vi "Scripting_ReplaceVisAndControls.vi"(0 "ViRef":refnum<vi>, 1 "OldVIsAndControls":path[](array[path]), 2 "NewVIsAndControls":path[](array[path]), 5 "error in (no error)":errorcluster) -> (15 "ReplacedVIsConPaneSize":u32[](array[numeric]), 19 "error out":errorcluster)   [LabVIEW 2012]
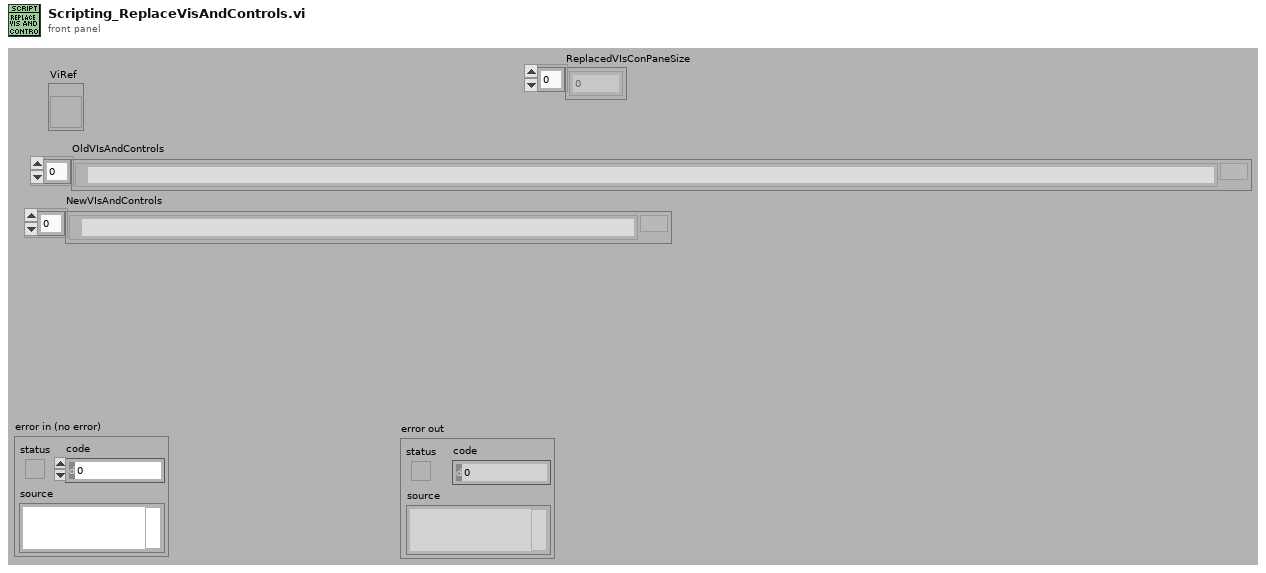
[diagram p1: front panel]
types:
  T1 = enum32{"invalid lock state", "Not Locked", "Locked (No Password)", "Password-protected"}
  T2 = cluster{"ClassControls":refnum<vi>[], "NewClassControl":path, "ReplacedVIsConPaneSize":u32[]}
  T3 = enum32{"not a typedef", "typedef", "strict typedef", "class private data"}
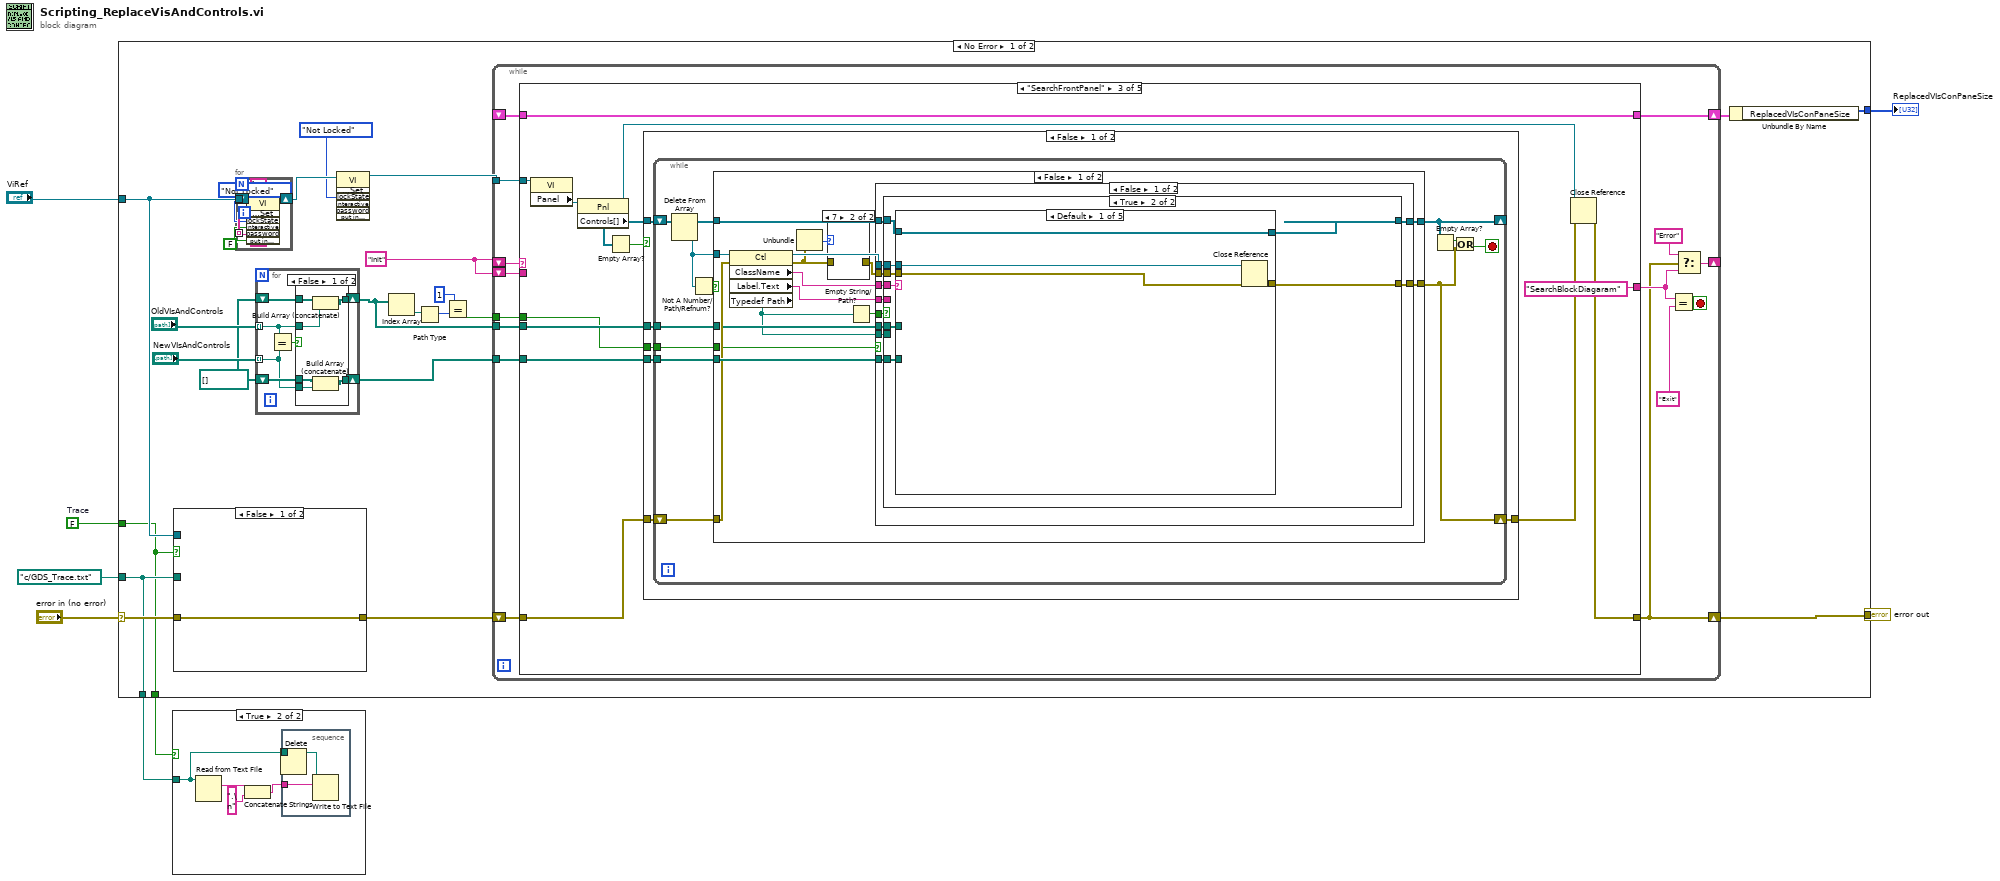
[diagram p0: block diagram]
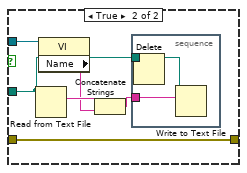
[diagram p3: hidden frame]
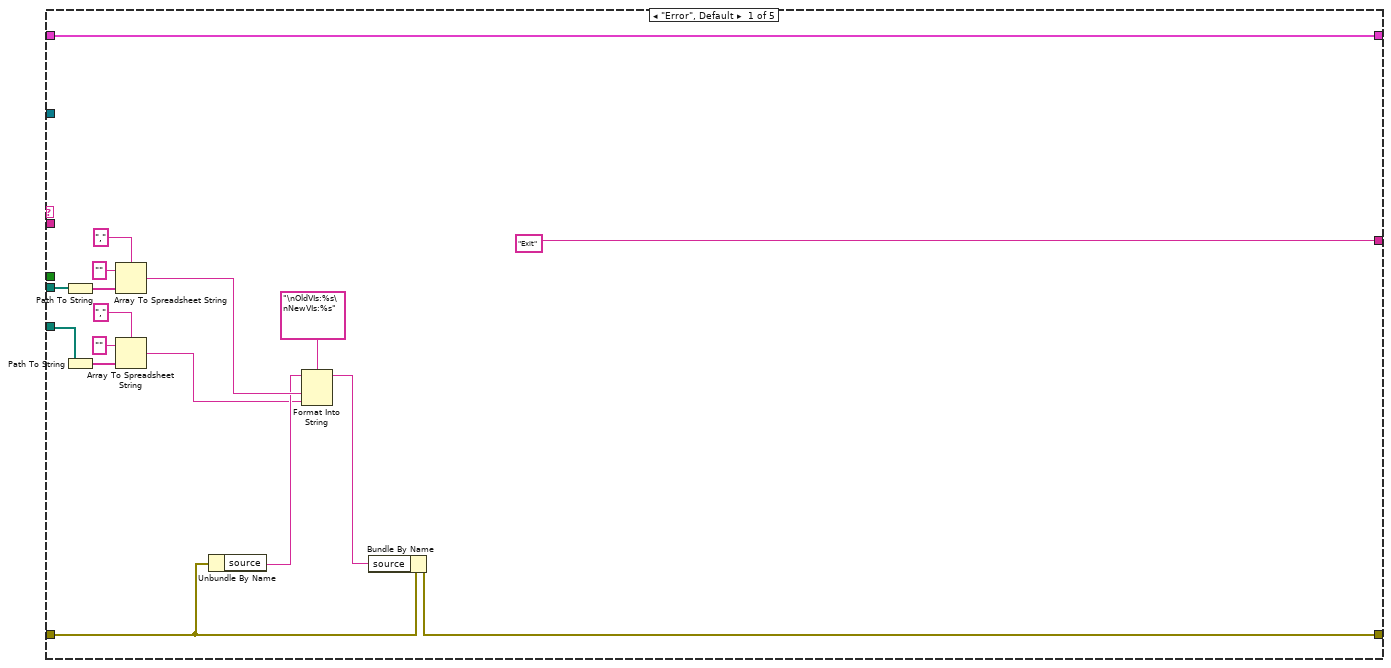
[diagram p5: hidden frame]
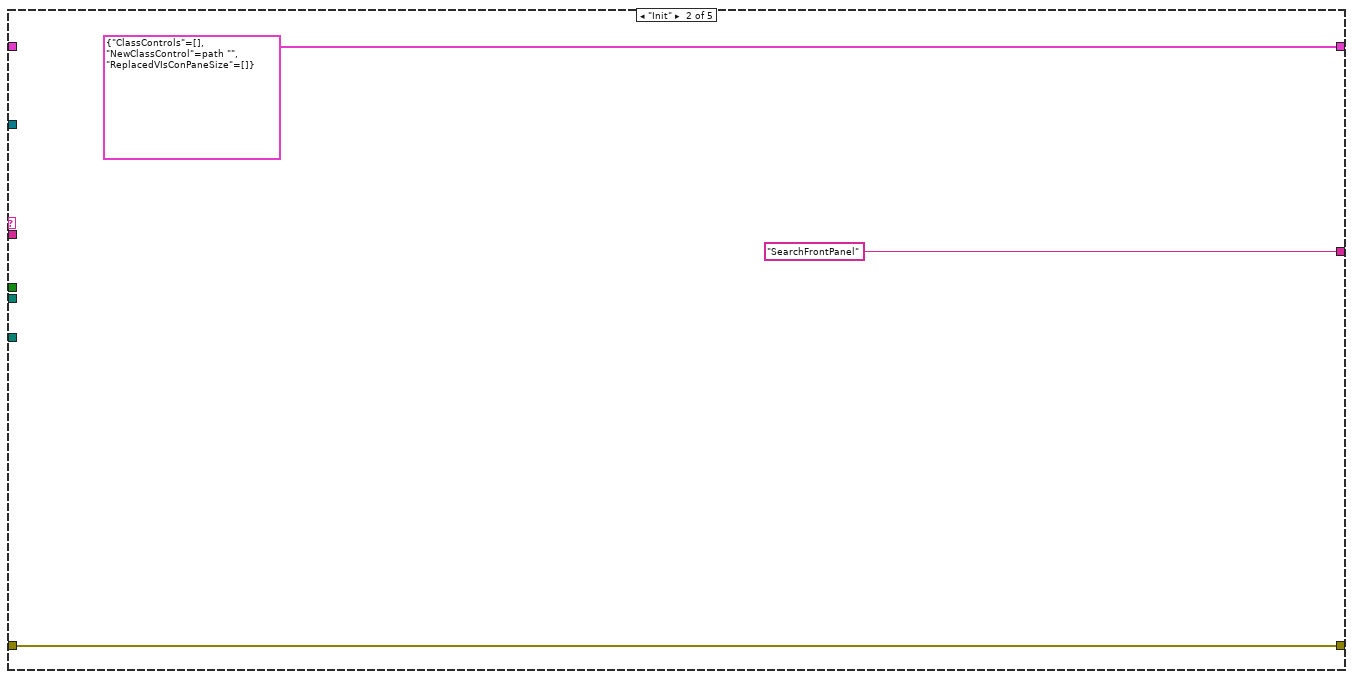
[diagram p6: hidden frame]
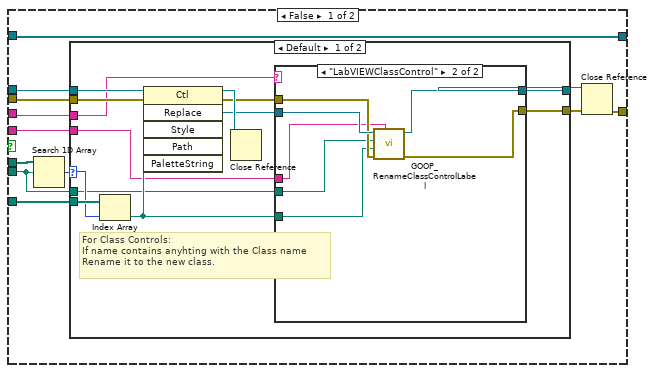
[diagram p8: hidden frame]
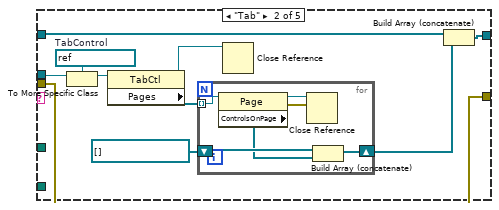
[diagram p11: hidden frame]
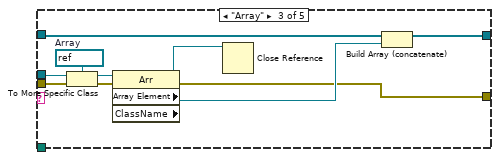
[diagram p12: hidden frame]
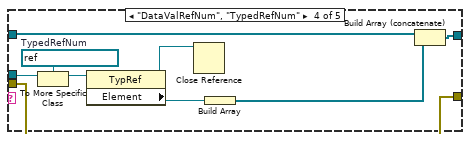
[diagram p13: hidden frame]
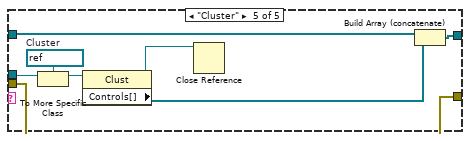
[diagram p14: hidden frame]
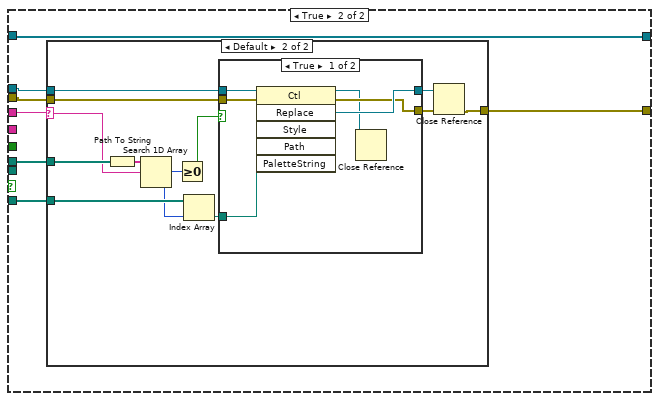
[diagram p15: hidden frame]
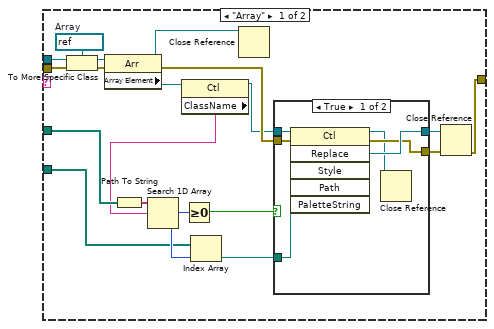
[diagram p16: hidden frame]
diagram:
  w6 = FALSE  # Trace
  n1 = case shown="No Error" "error in (no error)" {
    selector: "error in (no error)" -> [w22 w808]
    tunnel: [w30 w808] -> w8
    tunnel: "ViRef" -> [w20 _]
    tunnel: w6 -> [w18 _]
    tunnel: path "c:/GDS_Trace.txt" -> [w19 _]
    tunnel: [w19 _] -> w4
    tunnel: [w18 _] -> w3
    tunnel: [w10 _] -> w1
    frame No Error {
      w23 = path[] []
      w9 = "Init"
      n2 = case shown="False" w18 {
        tunnel: w22 -> [w31 w36]
        tunnel: [w31 w36] -> w21
        tunnel: w20 -> [_ w37]
        tunnel: w19 -> [_ w32]
        frame False {
        }
        frame True {
          n3 = Read from Text File(file (use dialog)=w32) -> (text=w35:string)  [unwired: 3 in, 3 out]
          n4 = property class="VI"(reference=w37) -> ("Name"=w34:string)  [unwired: 1 in, 2 out]
          n5 = Concatenate Strings(w35, w34) -> (w33:string)
          n6 = stacked-sequence {
            tunnel: w33 -> [w40]
            tunnel: w32 -> [w39]
            frame #0 {
              n7 = Delete(path (use dialog)=w39) -> (deleted path=w38:path)  [unwired: 4 in, 2 out]
              n8 = Write to Text File(file (use dialog)=w38, text=w40) -> ()  [unwired: 2 in, 3 out]
            }
          }
        }
      }
      n9 = for {
        tunnel: string[] ["goop rules", "i love goteborg", "Endevo Knows Goop!", "kiss"] -> [w58] mode=indexing
        shift-right: [w56] -> w28
        shift-left: w20 -> [_]
        tunnel: w20 -> [w57]
        w59 = FALSE ("Interactive")
        n10 = invoke class="VI" method="Lock State.Set"(reference=w57, "lockState"=T1."Not Locked" ("Lock State"), "interactive"=w59, "password"=w58, "put in Cache"=w59) -> (reference out=w56:refnum<vi>)  [unwired: 2 in, 6 out]
      }
      n11 = for {
        tunnel: "NewVIsAndControls" -> [w41] mode=indexing
        tunnel: "OldVIsAndControls" -> [w44] mode=indexing
        shift-right: [w45] -> w17
        shift-left: w23 -> [w46]
        shift-right: [w43] -> w13
        shift-left: w23 -> [w42]
        n12 = Equal?(x=w44, y=w41) -> (x = y?=w47:bool)
        n13 = case shown="False" w47 {
          tunnel: w46 -> [w53 w55]
          tunnel: [w52 w55] -> w45
          tunnel: w44 -> [w51 _]
          tunnel: w42 -> [w49 w54]
          tunnel: [w50 w54] -> w43
          tunnel: w41 -> [w48 _]
          frame False {
            n14 = Build Array (concatenate)(w53, w51) -> (w52:path[])
            n15 = Build Array (concatenate)(w49, w48) -> (w50:path[])
          }
          frame True {
          }
        }
      }
      n16 = invoke class="VI" method="Lock State.Set"(reference=w28, "lockState"=T1."Not Locked" ("Lock State")) -> (reference out=w26:refnum<vi>)  [unwired: 5 in, 6 out]
      n17 = Index Array(array=w17) -> (element=w14:path)  [unwired: 1 in]
      n18 = Path Type(1:w14) -> (0:w16:i16)
      n19 = Equal?(x=i16 1, y=w16) -> (x = y?=w12:bool)
      n20 = while {
        shift-right: [w68] -> w30
        shift-left: w21 -> [w75]
        shift-right: [w73] -> _
        shift-left: w9 -> [w74]
        shift-right: [w67] -> w11
        shift-left: _ -> [w66]
        tunnel: w26 -> [w63]
        tunnel: w17 -> [w65]
        tunnel: w13 -> [w64]
        tunnel: w12 -> [w62]
        shift-left: w9 -> [w61]
        stop <- w72 stop-if-true
        n21 = case shown="\"SearchFrontPanel\"" w74 {
          tunnel: w75 -> [w90 w95 w101 w310 w793]
          tunnel: [w89 w95 w100 w311 w792] -> w68
          tunnel: ["Exit" "SearchFrontPanel" "SearchBlockDiagaram" "Save" "Exit"] -> w69
          tunnel: [w91 T2 {"ClassControls"=[], "NewClassControl"=path "", "ReplacedVIsConPaneSize"=[]} w104 w304 w789] -> w67
          tunnel: w66 -> [w91 _ w104 w305 w789]
          tunnel: w63 -> [_ _ w108 w314 w794]
          tunnel: w65 -> [w88 _ w106 w309 _]
          tunnel: w64 -> [w78 _ w105 w308 _]
          tunnel: w62 -> [_ _ w96 w306 _]
          tunnel: w61 -> [_ _ _ _ _]
          frame "Error", Default {
            n22 = Path To String(path=w88) -> (string=w87:string[])
            n23 = Path To String(path=w78) -> (string=w79:string[])
            n24 = Array To Spreadsheet String(delimiter (Tab)=",", array=w87, 3:"" ("format string")) -> (spreadsheet string=w84:string)
            n25 = Array To Spreadsheet String(delimiter (Tab)=",", array=w79, 3:"" ("format string")) -> (spreadsheet string=w76:string)
            n26 = Unbundle By Name(w90) -> ("source"=w77:string)
            n27 = Format Into String(format string="\nOldVIs:%s\nNewVIs:%s", initial string=w77, w84, w76) -> (resulting string=w82:string)  [unwired: 1 in, 1 out]
            n28 = Bundle By Name(cluster=w90, "source"=w82) -> (w89:errorcluster)
          }
          frame "Init" {
          }
          frame "SearchFrontPanel" {
            n29 = property class="VI"(reference=w108) -> ("Panel"=w107:refnum<vi>)  [unwired: 1 in, 2 out]
            n30 = property class="Pnl"(reference=w107) -> (reference out=w99:refnum<vi>, "Controls[]"=w98:refnum<vi>[])  [unwired: 1 in, 1 out]
            n31 = Empty Array?(array=w98) -> (empty?=w97:bool)
            n32 = case shown="False" w97 {
              tunnel: w106 -> [w114 _]
              tunnel: w105 -> [w113 _]
              tunnel: [w112 w302] -> w102
              tunnel: w101 -> [w111 w302]
              tunnel: w98 -> [w110 _]
              tunnel: w96 -> [w109 _]
              frame False {
                n33 = while {
                  shift-right: [w118] -> _
                  shift-left: w110 -> [w126]
                  tunnel: w114 -> [w122]
                  tunnel: w113 -> [w124]
                  shift-right: [w115] -> w112
                  shift-left: w111 -> [w123]
                  tunnel: w109 -> [w119]
                  stop <- w116 stop-if-true
                  n34 = Delete From Array(array=w126) -> (deleted portion=w121:refnum<vi>, array with subset deleted=w125:refnum<vi>[])  [unwired: 2 in]
                  n35 = Not A Number/Path/Refnum?(number/path/refnum=w121) -> (NaN/Path/Refnum?=w120:bool)
                  n36 = case shown="False" w120 {
                    tunnel: w125 -> [w140 w300]
                    tunnel: [w139 w300] -> w118
                    tunnel: w124 -> [w138 _]
                    tunnel: w123 -> [w137 w301]
                    tunnel: [w136 w301] -> w115
                    tunnel: w122 -> [w135 _]
                    tunnel: w121 -> [w132 _]
                    tunnel: w119 -> [w131 _]
                    frame False {
                      n37 = property class="Ctl"(reference=w132, error in=w137) -> (reference out=w141:refnum<vi>, error out=w128:errorcluster, "ClassName"=w142:string, "Label.Text"=w130:string, "Typedef Path"=w134:path)
                      n38 = Unbundle(w128) -> ("code"=w129:i32)  [unwired: 2 out]
                      n39 = case shown="7" w129 {
                        tunnel: w128 -> [w143 _]
                        tunnel: [w143 _] -> w127
                        frame 0, Default {
                        }
                        frame 7 {
                        }
                      }
                      n40 = Empty String/Path?(string/path=w134) -> (empty?=w133:bool)
                      n41 = case shown="False" w131 {
                        tunnel: w142 -> [w154 w246]
                        tunnel: w141 -> [w153 w251]
                        tunnel: w140 -> [w152 w248]
                        tunnel: [w151 w248] -> w139
                        tunnel: w138 -> [w150 w249]
                        tunnel: w127 -> [w149 w250]
                        tunnel: [w148 w252] -> w136
                        tunnel: w135 -> [w147 w247]
                        tunnel: w134 -> [w146 _]
                        tunnel: w133 -> [w145 _]
                        tunnel: w130 -> [w144 _]
                        frame False {
                          n42 = case shown="True" w145 {
                            tunnel: w154 -> [w157 w198]
                            tunnel: w153 -> [w162 w197]
                            tunnel: w152 -> [w160 w196]
                            tunnel: [w160 w195] -> w151
                            tunnel: w150 -> [w163 w194]
                            tunnel: w149 -> [w161 w193]
                            tunnel: [w164 w192] -> w148
                            tunnel: w147 -> [w159 w191]
                            tunnel: w146 -> [w155 _]
                            tunnel: w144 -> [w156 _]
                            frame False {
                              n43 = Search 1D Array(1D array=w159, element=w155) -> (index of element=w158:i32)  [unwired: 1 in]
                              n44 = case shown="Default" w158 {
                                selector: w158 -> [w176 _]
                                tunnel: [w172 w190] -> w166
                                tunnel: [w170 w189] -> w165
                                tunnel: w163 -> [w178 _]
                                tunnel: w162 -> [w175 w190]
                                tunnel: w161 -> [w177 w189]
                                tunnel: w157 -> [w174 _]
                                tunnel: w156 -> [w167 _]
                                tunnel: w155 -> [w168 _]
                                frame Default {
                                # "For Class Controls:\nIf name contains anyhting with the Class name\nRename it to the new class."
                                n45 = Index Array(array=w178, index=w176) -> (element=w169:path)
                                n46 = invoke class="Ctl" method="Replace"(reference=w175, error in=w177, "Path"=w169) -> (reference out=w179:refnum<vi>, error out=w171:errorcluster, "Replace"=w173:refnum<vi>)  [unwired: 3 in, 3 out]
                                n47 = Close Reference(reference=w179) -> ()  [unwired: 1 in, 1 out]
                                n48 = case shown="\"LabVIEWClassControl\"" w174 {
                                tunnel: w173 -> [w181 w188]
                                tunnel: [w181 w187] -> w172
                                tunnel: w171 -> [w180 w185]
                                tunnel: [w180 w186] -> w170
                                tunnel: w169 -> [_ w184]
                                tunnel: w168 -> [_ w183]
                                tunnel: w167 -> [_ w182]
                                frame Default {
                                }
                                frame "LabVIEWClassControl" {
                                n49 = call <resource>:"GOOP_RenameClassControlLabel.vi"("Label.Text"=w182, "error in (no error)"=w185, "Path"=w184, "Typedef Path"=w183, "GObject in"=w188) -> ("error out"=w186:errorcluster, "Control out"=w187:refnum<vi>)  [unwired: 5 in]
                                }
                                }
                                }
                                frame -1 {
                                }
                              }
                              n50 = Close Reference(reference=w166, error in (no error)=w165) -> (error out=w164:errorcluster)
                            }
                            frame True {
                              n51 = case shown="Default" w198 {
                                tunnel: w197 -> [w200 w212 w228 w237 w245]
                                tunnel: w196 -> [w202 w207 w222 w234 w242]
                                tunnel: [w202 w205 w219 w233 w241] -> w195
                                tunnel: w194 -> [_ _ _ _ _]
                                tunnel: w193 -> [w199 w203 w223 w231 w239]
                                tunnel: [w201 w203 w220 w231 w239] -> w192
                                tunnel: w191 -> [_ _ _ _ _]
                                frame Default {
                                n52 = Close Reference(reference=w200, error in (no error)=w199) -> (error out=w201:errorcluster)
                                }
                                frame "Tab" {
                                w211 = refnum<vi> refnum  # TabControl
                                n53 = To More Specific Class(target class=w211, reference=w212) -> (specific class reference=w210:refnum<vi>)  [unwired: 1 in, 1 out]
                                n54 = property class="TabCtl"(reference=w210) -> (reference out=w204:refnum<vi>, "Pages"=w209:refnum<vi>[])  [unwired: 1 in, 1 out]
                                n55 = for {
                                tunnel: w209 -> [w218] mode=indexing
                                shift-right: [w217] -> w206
                                shift-left: refnum<vi>[] [] -> [w216]
                                n56 = property class="Page"(reference=w218) -> (reference out=w213:refnum<vi>, error out=w214:errorcluster, "ControlsOnPage"=w215:refnum<vi>[])  [unwired: 1 in]
                                n57 = Close Reference(reference=w213, error in (no error)=w214) -> ()  [unwired: 1 out]
                                n58 = Build Array (concatenate)(w216, w215) -> (w217:refnum<vi>[])
                                }
                                n59 = Close Reference(reference=w204) -> ()  [unwired: 1 in, 1 out]
                                n60 = Build Array (concatenate)(w207, w206) -> (w205:refnum<vi>[])
                                }
                                frame "Array" {
                                w227 = refnum<vi> refnum  # Array
                                n61 = To More Specific Class(target class=w227, reference=w228, error in=w223) -> (specific class reference=w226:refnum<vi>, error out=w224:errorcluster)
                                n62 = property class="Arr" props=["Array Element", "ClassName"](reference=w226, error in=w224) -> (reference out=w225:refnum<vi>, error out=w220:errorcluster, "Array Element"=w221:refnum<vi>)  [unwired: 1 out]
                                n63 = Close Reference(reference=w225) -> ()  [unwired: 1 in, 1 out]
                                n64 = Build Array (concatenate)(w222, w221) -> (w219:refnum<vi>[])
                                }
                                frame "DataValRefNum", "TypedRefNum" {
                                w236 = refnum<vi> refnum  # TypedRefNum
                                n65 = To More Specific Class(target class=w236, reference=w237) -> (specific class reference=w235:refnum<vi>)  [unwired: 1 in, 1 out]
                                n66 = property class="TypRef"(reference=w235) -> (reference out=w232:refnum<vi>, "Element"=w230:refnum<vi>)  [unwired: 1 in, 1 out]
                                n67 = Close Reference(reference=w232) -> ()  [unwired: 1 in, 1 out]
                                n68 = Build Array(w230) -> (w229:refnum<vi>[])
                                n69 = Build Array (concatenate)(w234, w229) -> (w233:refnum<vi>[])
                                }
                                frame "Cluster" {
                                w244 = refnum<vi> refnum  # Cluster
                                n70 = To More Specific Class(target class=w244, reference=w245) -> (specific class reference=w243:refnum<vi>)  [unwired: 1 in, 1 out]
                                n71 = property class="Clust"(reference=w243) -> (reference out=w240:refnum<vi>, "Controls[]"=w238:refnum<vi>[])  [unwired: 1 in, 1 out]
                                n72 = Close Reference(reference=w240) -> ()  [unwired: 1 in, 1 out]
                                n73 = Build Array (concatenate)(w242, w238) -> (w241:refnum<vi>[])
                                }
                              }
                            }
                          }
                        }
                        frame True {
                          n74 = case shown="Default" w246 {
                            selector: w246 -> [_ w280]
                            tunnel: [w256 w289] -> w252
                            tunnel: w251 -> [w259 w288]
                            tunnel: w250 -> [w260 w287]
                            tunnel: w249 -> [w258 w286]
                            tunnel: w247 -> [w257 w284]
                            frame "Array" {
                              w271 = refnum<vi> refnum  # Array
                              n75 = To More Specific Class(target class=w271, reference=w259, error in=w260) -> (specific class reference=w270:refnum<vi>, error out=w261:errorcluster)
                              n76 = property class="Arr"(reference=w270, error in=w261) -> (reference out=w269:refnum<vi>, error out=w262:errorcluster, "Array Element"=w255:refnum<vi>)
                              n77 = Path To String(path=w257) -> (string=w265:string[])
                              n78 = property class="Ctl"(reference=w255) -> (reference out=w254:refnum<vi>, "ClassName"=w253:string)  [unwired: 1 in, 1 out]
                              n79 = Search 1D Array(1D array=w265, element=w253) -> (index of element=w263:i32)  [unwired: 1 in]
                              n80 = Greater Or Equal To 0?(x=w263) -> (x >= 0?=w264:bool)
                              n81 = Index Array(array=w258, index=w263) -> (element=w266:path)
                              n82 = Close Reference(reference=w269) -> ()  [unwired: 1 in, 1 out]
                              n83 = case shown="True" w264 {
                                tunnel: [w277 w279] -> w268
                                tunnel: [w276 w278] -> w267
                                tunnel: w254 -> [w274 w279]
                                tunnel: w262 -> [w273 w278]
                                tunnel: w266 -> [w272 _]
                                frame True {
                                n84 = invoke class="Ctl" method="Replace"(reference=w274, error in=w273, "Path"=w272) -> (reference out=w275:refnum<vi>, error out=w276:errorcluster, "Replace"=w277:refnum<vi>)  [unwired: 3 in, 3 out]
                                n85 = Close Reference(reference=w275) -> ()  [unwired: 1 in, 1 out]
                                }
                                frame False {
                                }
                              }
                              n86 = Close Reference(reference=w268, error in (no error)=w267) -> (error out=w256:errorcluster)
                            }
                            frame Default {
                              n87 = Path To String(path=w284) -> (string=w283:string[])
                              n88 = Search 1D Array(1D array=w283, element=w280) -> (index of element=w281:i32)  [unwired: 1 in]
                              n89 = Greater Or Equal To 0?(x=w281) -> (x >= 0?=w282:bool)
                              n90 = Index Array(array=w286, index=w281) -> (element=w285:path)
                              n91 = case shown="True" w282 {
                                tunnel: [w297 w299] -> w291
                                tunnel: [w296 w298] -> w290
                                tunnel: w288 -> [w294 w299]
                                tunnel: w287 -> [w293 w298]
                                tunnel: w285 -> [w292 _]
                                frame True {
                                n92 = invoke class="Ctl" method="Replace"(reference=w294, error in=w293, "Path"=w292) -> (reference out=w295:refnum<vi>, error out=w296:errorcluster, "Replace"=w297:refnum<vi>)  [unwired: 3 in, 3 out]
                                n93 = Close Reference(reference=w295) -> ()  [unwired: 1 in, 1 out]
                                }
                                frame False {
                                }
                              }
                              n94 = Close Reference(reference=w291, error in (no error)=w290) -> (error out=w289:errorcluster)
                            }
                          }
                        }
                      }
                    }
                    frame True {
                    }
                  }
                  n95 = Empty Array?(array=w118) -> (empty?=w117:bool)
                  n96 = Or(x=w117, y=w115) -> (x .or. y?=w116:bool)
                }
              }
              frame True {
              }
            }
            n97 = Close Reference(reference=w99, error in (no error)=w102) -> (error out=w100:errorcluster)
          }
          frame "SearchBlockDiagaram" {
            n98 = property class="VI"(reference=w314) -> (error out=w307:errorcluster, "Diagram"=w313:refnum<vi>)  [unwired: 1 in, 1 out]
            n99 = case shown="No Error" w307 {
              tunnel: w313 -> [w324 w787]
              tunnel: [w322 w788] -> w311
              tunnel: w310 -> [w321 w788]
              tunnel: w309 -> [w320 _]
              tunnel: w308 -> [w319 _]
              tunnel: w306 -> [w317 _]
              tunnel: [w315 _] -> w303
              frame No Error {
                n100 = property class="TopLvlDiag"(reference=w324) -> (reference out=w318:refnum<vi>, "AllObjs[]"=w323:refnum<vi>[])  [unwired: 1 in, 1 out]
                n101 = while {
                  shift-right: [w337] -> _
                  shift-left: w323 -> [w341]
                  shift-right: [w326] -> w322
                  shift-left: w321 -> [w335]
                  tunnel: w320 -> [w334]
                  tunnel: w319 -> [w333]
                  tunnel: w317 -> [w330]
                  shift-right: [w328] -> w315
                  shift-left: u32[] [] -> [w329]
                  stop <- w339 stop-if-true
                  # "LabVIEWClassConstant"
                  n102 = Delete From Array(array=w341) -> (deleted portion=w332:refnum<vi>, array with subset deleted=w338:refnum<vi>[])  [unwired: 2 in]
                  n103 = Not A Number/Path/Refnum?(number/path/refnum=w332) -> (NaN/Path/Refnum?=w331:bool)
                  n104 = case shown="False" w331 {
                    tunnel: [w355 _] -> w336
                    tunnel: [w352 w786] -> w327
                    tunnel: w335 -> [w351 w786]
                    tunnel: w334 -> [w350 _]
                    tunnel: w333 -> [w349 _]
                    tunnel: w332 -> [w348 _]
                    tunnel: w330 -> [w347 _]
                    tunnel: w329 -> [w346 w785]
                    tunnel: [w345 w785] -> w328
                    frame False {
                      n105 = property class="GObj"(reference=w348, error in=w351) -> (reference out=w357:refnum<vi>, error out=w358:errorcluster, "Class Name"=w356:string)
                      n106 = case shown="False" w347 {
                        tunnel: w358 -> [w368 w735]
                        tunnel: w357 -> [w367 w738]
                        tunnel: w356 -> [w366 w732]
                        tunnel: [w365 _] -> w355
                        tunnel: [w364 w736] -> w354
                        tunnel: [w363 w737] -> w353
                        tunnel: w350 -> [w362 w733]
                        tunnel: w349 -> [w361 w739]
                        tunnel: w346 -> [w360 w731]
                        tunnel: [w359 w731] -> w345
                        frame False {
                          n107 = case shown="Default" w366 {
                            selector: w366 -> [w378 _ _ _ _ _ _ _ _ _]
                            tunnel: w367 -> [w376 w589 w609 w629 w649 w669 w688 w707 w718 w730]
                            tunnel: w368 -> [w377 w584 w604 w626 w646 w666 w687 w703 w714 w726]
                            tunnel: [w371 w582 w602 w619 w640 w662 w680 w699 w710 w721] -> w364
                            tunnel: [w372 w580 w600 w621 w641 w660 w679 w701 w712 w724] -> w365
                            tunnel: [w373 w583 w603 w620 w639 w661 w681 w700 w711 w723] -> w363
                            tunnel: w362 -> [w375 _ _ _ _ _ _ _ _ _]
                            tunnel: w361 -> [w374 _ _ _ _ _ _ _ _ _]
                            tunnel: w360 -> [w370 w578 w598 w618 w638 w658 w678 w697 w708 w719]
                            tunnel: [w369 w578 w598 w618 w638 w658 w678 w697 w708 w719] -> w359
                            frame Default {
                              n108 = case shown="\"PolymorphicSubVI\", \"SubVI\"" w378 {
                                selector: w378 -> [w380 _ _ _ _]
                                tunnel: w377 -> [w383 w467 w503 w522 w555]
                                tunnel: w376 -> [w385 w468 w504 w532 w564]
                                tunnel: [w387 w466 w502 w531 w563] -> w371
                                tunnel: [w384 w465 w501 w530 w562] -> w373
                                tunnel: w375 -> [w382 w459 w495 w526 w558]
                                tunnel: w374 -> [w381 w456 w492 w523 w556]
                                tunnel: [_ _ _ w515 w547] -> w372
                                tunnel: w370 -> [w379 w455 w491 w514 w546]
                                tunnel: [w379 w454 w491 w514 w546] -> w369
                                frame Default {
                                w389 = refnum<vi> refnum  # Constant
                                n109 = To More Specific Class(target class=w389, reference=w385, error in=w383) -> (specific class reference=w388:refnum<vi>, error out=w386:errorcluster)
                                n110 = case shown="Error" w386 {
                                selector: w386 -> [w399 _]
                                tunnel: w388 -> [w395 _]
                                tunnel: [w400 w452] -> w387
                                tunnel: w385 -> [w393 w453]
                                tunnel: [w398 w453] -> w384
                                tunnel: w383 -> [w394 w452]
                                tunnel: w382 -> [w392 _]
                                tunnel: w381 -> [w390 _]
                                tunnel: w380 -> [w396 _]
                                frame No Error {
                                n111 = case shown="Default" w396 {
                                tunnel: w395 -> [_ w447]
                                tunnel: w399 -> [w419 w446]
                                tunnel: [w412 w445] -> w397
                                tunnel: w393 -> [w420 _]
                                tunnel: w392 -> [w418 w444]
                                tunnel: [w413 w443] -> w391
                                frame "LabVIEWClassConstant" {
                                w421 = refnum<vi> refnum  # LabVIEWClassConstant
                                n112 = for {
                                tunnel: w418 -> [w440] mode=indexing
                                tunnel: [w439] -> w417 mode=indexing
                                n113 = Strip Path(path=w440) -> (name=w439:string)  [unwired: 1 out]
                                }
                                n114 = To More Specific Class(target class=w421, reference=w420, error in=w419) -> (specific class reference=w423:refnum<vi>, error out=w422:errorcluster)
                                n115 = disable-structure shown="Enabled" {
                                disable-tunnel: w423 -> [w430 _]
                                disable-tunnel: w422 -> [w429 w438]
                                disable-tunnel: [w428 "-1"] -> w414
                                disable-tunnel: [w424 w438] -> w412
                                frame Enabled {
                                n116 = property class="LVClassConstant"(reference=w430, error in=w429) -> (error out=w424:errorcluster, "Value"=w431:variant)  [unwired: 1 out]
                                n117 = Flatten To String(anything=w431) -> (data string=w432:string)  [unwired: 3 in, 2 out]
                                n118 = Match Pattern(string=w432, regular expression="[~\\00\\01\\02\\03\\04\\05\\06\\07\\08\\09\\0A\\0B\\0C\\0D\\0E\\0F\\10\\11\\12\\13\\14\\15\\16\\17\\18\\19\\1A\\1B\\1C\\1D\\1E]+\\.lvclass") -> (match substring=w426:string)  [unwired: 1 in, 3 out]
                                n119 = Match Pattern(string=w426, regular expression="[~A-Za-zäöåÄÖÅÜü_]*") -> (after substring=w425:string)  [unwired: 1 in, 3 out]
                                n120 = Match Pattern(string=w425, regular expression="\\.lvclass") -> (before substring=w436:string)  [unwired: 1 in, 3 out]
                                n121 = Format Into String(format string="%s.ctl", w436) -> (resulting string=w428:string)  [unwired: 2 in, 1 out]
                                }
                                frame Disabled {
                                }
                                }
                                n122 = To Lower Case(string=w417) -> (all lower case string=w416:string[])
                                n123 = To Lower Case(string=w414) -> (all lower case string=w415:string)
                                n124 = Search 1D Array(1D array=w416, element=w415) -> (index of element=w413:i32)  [unwired: 1 in]
                                }
                                frame Default {
                                n125 = property class="Const"(reference=w447, error in=w446) -> (error out=w445:errorcluster, "Typedef Path"=w442:path)  [unwired: 1 out]
                                n126 = Empty String/Path?(string/path=w442) -> (empty?=w441:bool)
                                n127 = case shown="False" w441 {
                                tunnel: w444 -> [w450 _]
                                tunnel: [w449 -1 ("index of element")] -> w443
                                tunnel: w442 -> [w448 _]
                                frame False {
                                n128 = Search 1D Array(1D array=w450, element=w448) -> (index of element=w449:i32)  [unwired: 1 in]
                                }
                                frame True {
                                }
                                }
                                }
                                }
                                n129 = case shown="0, Default" w391 {
                                selector: w391 -> [w407 _]
                                tunnel: w394 -> [w408 w410]
                                tunnel: w395 -> [w409 w411]
                                tunnel: [w403 w411] -> w398
                                tunnel: [w402 w410] -> w400
                                tunnel: w390 -> [w406 _]
                                tunnel: w397 -> [_ _]
                                tunnel: [w401 _] -> _
                                frame 0, Default {
                                n130 = Index Array(array=w406, index=w407) -> (element=w405:path)
                                n131 = invoke class="Const" method="Replace"(reference=w409, error in=w408, "Path"=w405) -> (reference out=w404:refnum<vi>, error out=w402:errorcluster, "Replace"=w403:refnum<vi>)  [unwired: 3 in, 3 out]
                                n132 = Close Reference(reference=w404) -> (error out=w401:errorcluster)  [unwired: 1 in]
                                }
                                frame -1 {
                                }
                                }
                                }
                                frame Error {
                                }
                                }
                                }
                                frame "PolymorphicSubVI", "SubVI" {
                                n133 = To More Specific Class(target class=refnum<vi> refnum ("WhileLoop"), reference=w468, error in=w467) -> (specific class reference=w463:refnum<vi>, error out=w462:errorcluster)
                                n134 = property class="SubVI"(reference=w463, error in=w462) -> (reference out=w460:refnum<vi>, error out=w461:errorcluster, "VI Path"=w458:path)
                                n135 = Search 1D Array(1D array=w459, element=w458) -> (index of element=w457:i32)  [unwired: 1 in]
                                n136 = case shown="0, Default" w457 {
                                selector: w457 -> [w487 _]
                                tunnel: w461 -> [w484 w489]
                                tunnel: w460 -> [w485 w490]
                                tunnel: [w480 w490] -> w465
                                tunnel: [w479 w489] -> w466
                                tunnel: w456 -> [w486 _]
                                tunnel: [w473 _] -> _
                                tunnel: w455 -> [w471 w488]
                                tunnel: [w469 w488] -> w454
                                frame 0, Default {
                                n137 = Index Array(array=w486, index=w487) -> (element=w483:path)
                                n138 = call <resource>:"Scripting_ReplaceSubVI.vi"("error in"=w484, "NewVIToReplaceWith"=w483, "CurrentSubVI"=w485) -> ("error out"=w479:errorcluster, "ReplacedObject(SubVI)"=w480:refnum<vi>)  [unwired: 7 in]
                                n139 = To More Specific Class(target class=refnum<vi> refnum ("WhileLoop"), reference=w480, error in=w479) -> (specific class reference=w478:refnum<vi>, error out=w477:errorcluster)
                                n140 = property class="SubVI"(reference=w478, error in=w477) -> ("VI Ref"=w476:refnum<vi>)  [unwired: 2 out]
                                n141 = property class="VI" props=["Exec.State", "ConPane"](reference=w476) -> (reference out=w472:refnum<vi>, "ConPane"=w482:refnum<vi>)  [unwired: 1 in, 2 out]
                                n142 = property class="ConPane"(reference=w482) -> (reference out=w474:refnum<vi>, error out=w475:errorcluster, "NumConns"=w470:u32)  [unwired: 1 in]
                                n143 = Build Array (concatenate)(w471, w470) -> (w469:u32[])
                                n144 = Close Reference(reference=w474, error in (no error)=w475) -> (error out=w473:errorcluster)
                                n145 = Close Reference(reference=w472, error in (no error)=w473) -> ()  [unwired: 1 out]
                                }
                                frame -1 {
                                }
                                }
                                }
                                frame "StaticVIReference" {
                                n146 = To More Specific Class(target class=refnum<vi> refnum ("WhileLoop"), reference=w504, error in=w503) -> (specific class reference=w499:refnum<vi>, error out=w498:errorcluster)
                                n147 = property class="StatVIRef"(reference=w499, error in=w498) -> (reference out=w496:refnum<vi>, error out=w497:errorcluster, "Path"=w494:path)
                                n148 = Search 1D Array(1D array=w495, element=w494) -> (index of element=w493:i32)  [unwired: 1 in]
                                n149 = case shown="-1" w493 {
                                selector: w493 -> [w511 _]
                                tunnel: w497 -> [w508 w512]
                                tunnel: w496 -> [w509 w513]
                                tunnel: [w506 w513] -> w501
                                tunnel: [w505 w512] -> w502
                                tunnel: w492 -> [w510 _]
                                frame 0, Default {
                                n150 = Index Array(array=w510, index=w511) -> (element=w507:path)
                                n151 = property class="StatVIRef"(reference=w509, error in=w508, "Path"=w507) -> (reference out=w506:refnum<vi>, error out=w505:errorcluster)
                                }
                                frame -1 {
                                }
                                }
                                }
                                frame "ClusterConstant" {
                                n152 = To More Specific Class(target class=refnum<vi> refnum ("WhileLoop"), reference=w532, error in=w522) -> (specific class reference=w528:refnum<vi>, error out=w527:errorcluster)
                                n153 = property class="ClustCnst"(reference=w528, error in=w527) -> (reference out=w520:refnum<vi>, error out=w519:errorcluster, "Typedef Path"=w525:path)
                                n154 = Search 1D Array(1D array=w526, element=w525) -> (index of element=w524:i32)  [unwired: 1 in]
                                n155 = property class="ClustCnst"(reference=w520, error in=w519) -> (reference out=w518:refnum<vi>, "Elements[]"=w516:refnum<vi>[], "Typedef?"=w521:T3)  [unwired: 1 out]
                                n156 = Not Equal To 0?(x=w521) -> (x != 0?=w517:bool)
                                n157 = case shown="True" w517 {
                                tunnel: [w533 _] -> w515
                                tunnel: w516 -> [w533 w534]
                                frame False {
                                }
                                frame True {
                                n158 = for {
                                tunnel: w534 -> [w535] mode=indexing
                                n159 = Close Reference(reference=w535) -> ()  [unwired: 1 in, 1 out]
                                }
                                }
                                }
                                n160 = case shown="0, Default" w524 {
                                selector: w524 -> [w541 _]
                                tunnel: w522 -> [w542 w544]
                                tunnel: w518 -> [w543 w545]
                                tunnel: [w537 w545] -> w530
                                tunnel: [w536 w544] -> w531
                                tunnel: w523 -> [w540 _]
                                frame 0, Default {
                                n161 = Index Array(array=w540, index=w541) -> (element=w539:path)
                                n162 = invoke class="ClustCnst" method="Replace"(reference=w543, error in=w542, "Path"=w539) -> (reference out=w538:refnum<vi>, error out=w536:errorcluster, "Replace"=w537:refnum<vi>)  [unwired: 3 in, 3 out]
                                n163 = Close Reference(reference=w538) -> ()  [unwired: 1 in, 1 out]
                                }
                                frame -1 {
                                }
                                }
                                }
                                frame "ArrayConstant" {
                                n164 = To More Specific Class(target class=refnum<vi> refnum ("WhileLoop"), reference=w564, error in=w555) -> (specific class reference=w560:refnum<vi>, error out=w559:errorcluster)
                                n165 = property class="ArrCnst"(reference=w560, error in=w559) -> (reference out=w550:refnum<vi>, error out=w551:errorcluster, "Typedef Path"=w557:path)
                                n166 = Search 1D Array(1D array=w558, element=w557) -> (index of element=w548:i32)  [unwired: 1 in]
                                n167 = property class="ArrCnst"(reference=w550, error in=w551) -> (reference out=w549:refnum<vi>, "Element"=w552:refnum<vi>, "Typedef?"=w554:T3)  [unwired: 1 out]
                                n168 = Not Equal To 0?(x=w554) -> (x != 0?=w553:bool)
                                n169 = case shown="False" w553 {
                                tunnel: w552 -> [w566 w567]
                                tunnel: [w565 _] -> w547
                                frame False {
                                n170 = Build Array(w566) -> (w565:refnum<vi>[])
                                }
                                frame True {
                                n171 = Close Reference(reference=w567) -> ()  [unwired: 1 in, 1 out]
                                }
                                }
                                n172 = case shown="0, Default" w548 {
                                selector: w548 -> [w573 _]
                                tunnel: w555 -> [w574 w576]
                                tunnel: w549 -> [w575 w577]
                                tunnel: [w569 w577] -> w562
                                tunnel: [w568 w576] -> w563
                                tunnel: w556 -> [w572 _]
                                frame 0, Default {
                                n173 = Index Array(array=w572, index=w573) -> (element=w571:path)
                                n174 = invoke class="ArrCnst" method="Replace"(reference=w575, error in=w574, "Path"=w571) -> (reference out=w570:refnum<vi>, error out=w568:errorcluster, "Replace"=w569:refnum<vi>)  [unwired: 3 in, 3 out]
                                n175 = Close Reference(reference=w570) -> ()  [unwired: 1 in, 1 out]
                                }
                                frame -1 {
                                }
                                }
                                }
                              }
                            }
                            frame "CaseSelector", "CaseStructure" {
                              n176 = To More Specific Class(target class=refnum<vi> refnum ("CaseSelector"), reference=w589, error in=w584) -> (specific class reference=w587:refnum<vi>, error out=w585:errorcluster)
                              n177 = property class="CaseSel"(reference=w587, error in=w585) -> (reference out=w583:refnum<vi>, error out=w581:errorcluster, "Frames[]"=w586:refnum<vi>[])
                              n178 = for {
                                tunnel: w586 -> [w597] mode=indexing
                                shift-right: [w590] -> w582
                                shift-left: w581 -> [w596]
                                shift-right: [w593] -> w580
                                shift-left: refnum<vi>[] [] -> [w595]
                                n179 = property class="Diag"(reference=w597, error in=w596) -> (reference out=w591:refnum<vi>, error out=w592:errorcluster, "AllObjs[]"=w594:refnum<vi>[])
                                n180 = Build Array (concatenate)(w595, w594) -> (w593:refnum<vi>[])
                                n181 = Close Reference(reference=w591, error in (no error)=w592) -> (error out=w590:errorcluster)
                              }
                            }
                            frame "DisableStructure" {
                              n182 = To More Specific Class(target class=refnum<vi> refnum ("CaseSelector"), reference=w609, error in=w604) -> (specific class reference=w607:refnum<vi>, error out=w605:errorcluster)
                              n183 = property class="DisableStructure"(reference=w607, error in=w605) -> (reference out=w603:refnum<vi>, error out=w601:errorcluster, "Frames[]"=w606:refnum<vi>[])
                              n184 = for {
                                tunnel: w606 -> [w617] mode=indexing
                                shift-right: [w610] -> w602
                                shift-left: w601 -> [w616]
                                shift-right: [w613] -> w600
                                shift-left: refnum<vi>[] [] -> [w615]
                                n185 = property class="Diag"(reference=w617, error in=w616) -> (reference out=w611:refnum<vi>, error out=w612:errorcluster, "AllObjs[]"=w614:refnum<vi>[])
                                n186 = Build Array (concatenate)(w615, w614) -> (w613:refnum<vi>[])
                                n187 = Close Reference(reference=w611, error in (no error)=w612) -> (error out=w610:errorcluster)
                              }
                            }
                            frame "MultiFrameStructure" {
                              (unwired) string[] []
                              n188 = To More Specific Class(target class=refnum<vi> refnum ("MultiFrameStructure"), reference=w629, error in=w626) -> (specific class reference=w628:refnum<vi>, error out=w627:errorcluster)
                              n189 = property class="MFStruct"(reference=w628, error in=w627) -> (reference out=w620:refnum<vi>, error out=w623:errorcluster, "Frames[]"=w622:refnum<vi>[])
                              n190 = for {
                                tunnel: w622 -> [w637] mode=indexing
                                shift-right: [w630] -> w619
                                shift-left: w623 -> [w636]
                                shift-right: [w633] -> w621
                                shift-left: refnum<vi>[] [] -> [w635]
                                n191 = property class="Diag"(reference=w637, error in=w636) -> (reference out=w631:refnum<vi>, error out=w632:errorcluster, "AllObjs[]"=w634:refnum<vi>[])
                                n192 = Build Array (concatenate)(w635, w634) -> (w633:refnum<vi>[])
                                n193 = Close Reference(reference=w631, error in (no error)=w632) -> (error out=w630:errorcluster)
                              }
                            }
                            frame "EventStructure" {
                              n194 = To More Specific Class(target class=refnum<vi> refnum ("EventStructure"), reference=w649, error in=w646) -> (specific class reference=w648:refnum<vi>, error out=w647:errorcluster)
                              n195 = property class="EvntStruct"(reference=w648, error in=w647) -> (reference out=w639:refnum<vi>, error out=w643:errorcluster, "Frames[]"=w642:refnum<vi>[])
                              n196 = for {
                                tunnel: w642 -> [w657] mode=indexing
                                shift-right: [w650] -> w640
                                shift-left: w643 -> [w656]
                                shift-right: [w653] -> w641
                                shift-left: refnum<vi>[] [] -> [w655]
                                n197 = property class="Diag"(reference=w657, error in=w656) -> (reference out=w651:refnum<vi>, error out=w652:errorcluster, "AllObjs[]"=w654:refnum<vi>[])
                                n198 = Build Array (concatenate)(w655, w654) -> (w653:refnum<vi>[])
                                n199 = Close Reference(reference=w651, error in (no error)=w652) -> (error out=w650:errorcluster)
                              }
                            }
                            frame "Sequence" {
                              n200 = To More Specific Class(target class=refnum<vi> refnum ("Sequence"), reference=w669, error in=w666) -> (specific class reference=w668:refnum<vi>, error out=w667:errorcluster)
                              n201 = property class="Seq"(reference=w668, error in=w667) -> (reference out=w661:refnum<vi>, error out=w663:errorcluster, "Frames[]"=w659:refnum<vi>[])
                              n202 = for {
                                tunnel: w659 -> [w677] mode=indexing
                                shift-right: [w670] -> w662
                                shift-left: w663 -> [w676]
                                shift-right: [w673] -> w660
                                shift-left: refnum<vi>[] [] -> [w675]
                                n203 = property class="Diag"(reference=w677, error in=w676) -> (reference out=w671:refnum<vi>, error out=w672:errorcluster, "AllObjs[]"=w674:refnum<vi>[])
                                n204 = Build Array (concatenate)(w675, w674) -> (w673:refnum<vi>[])
                                n205 = Close Reference(reference=w671, error in (no error)=w672) -> (error out=w670:errorcluster)
                              }
                            }
                            frame "FlatSequence" {
                              n206 = To More Specific Class(target class=refnum<vi> refnum ("FlatSequence"), reference=w688, error in=w687) -> (specific class reference=w685:refnum<vi>)  [unwired: 1 out]
                              n207 = property class="FlatSeq"(reference=w685) -> (reference out=w681:refnum<vi>, error out=w683:errorcluster, "Diagrams[]"=w682:refnum<vi>[])  [unwired: 1 in]
                              n208 = for {
                                tunnel: w682 -> [w696] mode=indexing
                                shift-right: [w689] -> w680
                                shift-left: w683 -> [w695]
                                shift-right: [w692] -> w679
                                shift-left: refnum<vi>[] [] -> [w694]
                                n209 = property class="Diag"(reference=w696, error in=w695) -> (reference out=w690:refnum<vi>, error out=w691:errorcluster, "AllObjs[]"=w693:refnum<vi>[])
                                n210 = Build Array (concatenate)(w694, w693) -> (w692:refnum<vi>[])
                                n211 = Close Reference(reference=w690, error in (no error)=w691) -> (error out=w689:errorcluster)
                              }
                            }
                            frame "WhileLoop" {
                              n212 = To More Specific Class(target class=refnum<vi> refnum ("WhileLoop"), reference=w707, error in=w703) -> (specific class reference=w706:refnum<vi>, error out=w704:errorcluster)
                              n213 = property class="WLoop"(reference=w706, error in=w704) -> (reference out=w700:refnum<vi>, error out=w699:errorcluster, "Diagram"=w702:refnum<vi>)
                              n214 = property class="Diag"(reference=w702) -> (reference out=w698:refnum<vi>, "AllObjs[]"=w701:refnum<vi>[])  [unwired: 1 in, 1 out]
                              n215 = Close Reference(reference=w698) -> ()  [unwired: 1 in, 1 out]
                            }
                            frame "TimedLoop" {
                              n216 = To More Specific Class(target class=refnum<vi> refnum ("WhileLoop"), reference=w718, error in=w714) -> (specific class reference=w717:refnum<vi>, error out=w715:errorcluster)
                              n217 = property class="WLoop"(reference=w717, error in=w715) -> (reference out=w711:refnum<vi>, error out=w710:errorcluster, "Diagram"=w713:refnum<vi>)
                              n218 = property class="Diag"(reference=w713) -> (reference out=w709:refnum<vi>, "AllObjs[]"=w712:refnum<vi>[])  [unwired: 1 in, 1 out]
                              n219 = Close Reference(reference=w709) -> ()  [unwired: 1 in, 1 out]
                            }
                            frame "ForLoop" {
                              n220 = To More Specific Class(target class=refnum<vi> refnum ("WhileLoop"), reference=w730, error in=w726) -> (specific class reference=w729:refnum<vi>, error out=w727:errorcluster)
                              n221 = property class="FLoop"(reference=w729, error in=w727) -> (reference out=w723:refnum<vi>, error out=w722:errorcluster, "Diagram"=w725:refnum<vi>)
                              n222 = property class="Diag"(reference=w725, error in=w722) -> (reference out=w720:refnum<vi>, error out=w721:errorcluster, "AllObjs[]"=w724:refnum<vi>[])
                              n223 = Close Reference(reference=w720, error in (no error)=w721) -> ()  [unwired: 1 out]
                            }
                          }
                        }
                        frame True {
                          n224 = Path To String(path=w733) -> (string=w734:string[])
                          n225 = case shown="Default" w732 {
                            selector: w732 -> [_ w767]
                            tunnel: w739 -> [w744 w776]
                            tunnel: w738 -> [w756 w775]
                            tunnel: [w750 w773] -> w737
                            tunnel: [w749 w772] -> w736
                            tunnel: w735 -> [w757 w771]
                            tunnel: w734 -> [w748 w770]
                            frame "ArrayConstant" {
                              n226 = To More Specific Class(target class=refnum<vi> refnum ("WhileLoop"), reference=w756, error in=w757) -> (specific class reference=w755:refnum<vi>, error out=w754:errorcluster)
                              n227 = property class="ArrCnst"(reference=w755, error in=w754) -> (reference out=w742:refnum<vi>, error out=w741:errorcluster, "Element"=w747:refnum<vi>)
                              n228 = property class="Const"(reference=w747, error in=w741) -> (reference out=w746:refnum<vi>, error out=w743:errorcluster, "Class Name"=w745:string)
                              n229 = Search 1D Array(1D array=w748, element=w745) -> (index of element=w751:i32)  [unwired: 1 in]
                              n230 = Close Reference(reference=w742, error in (no error)=w743) -> (error out=w740:errorcluster)
                              n231 = Greater Or Equal To 0?(x=w751) -> (x >= 0?=w752:bool)
                              n232 = Index Array(array=w744, index=w751) -> (element=w753:path)
                              n233 = case shown="True" w752 {
                                tunnel: w746 -> [w760 w766]
                                tunnel: w753 -> [_ w765]
                                tunnel: [w760 w762] -> w750
                                tunnel: [w759 w764] -> w749
                                tunnel: w740 -> [w759 w763]
                                frame False {
                                }
                                frame True {
                                n234 = invoke class="Const" method="Replace"(reference=w766, error in=w763, "Path"=w765) -> (reference out=w761:refnum<vi>, error out=w764:errorcluster, "Replace"=w762:refnum<vi>)  [unwired: 3 in, 3 out]
                                n235 = Close Reference(reference=w761) -> ()  [unwired: 1 in, 1 out]
                                }
                              }
                            }
                            frame Default {
                              n236 = Search 1D Array(1D array=w770, element=w767) -> (index of element=w768:i32)  [unwired: 1 in]
                              n237 = Greater Or Equal To 0?(x=w768) -> (x >= 0?=w769:bool)
                              n238 = Index Array(array=w776, index=w768) -> (element=w774:path)
                              n239 = case shown="True" w769 {
                                tunnel: w775 -> [w778 w784]
                                tunnel: w774 -> [_ w783]
                                tunnel: [w778 w780] -> w773
                                tunnel: [w777 w782] -> w772
                                tunnel: w771 -> [w777 w781]
                                frame False {
                                }
                                frame True {
                                n240 = invoke class="GObj" method="Replace"(reference=w784, error in=w781, "Path"=w783) -> (reference out=w779:refnum<vi>, error out=w782:errorcluster, "Replace"=w780:refnum<vi>)  [unwired: 3 in, 3 out]
                                n241 = Close Reference(reference=w779) -> ()  [unwired: 1 in, 1 out]
                                }
                              }
                            }
                          }
                        }
                      }
                      n242 = Close Reference(reference=w353, error in (no error)=w354) -> (error out=w352:errorcluster)
                    }
                    frame True {
                    }
                  }
                  n243 = Build Array (concatenate)(w338, w336) -> (w337:refnum<vi>[])
                  n244 = Array Size(array=w337) -> (size(s)=w340:i32)
                  n245 = Equal To 0?(x=w340) -> (x = 0?=w339:bool)
                  n246 = Unbundle(w327) -> ("code"=w325:i32)  [unwired: 2 out]
                  n247 = case shown="0, Default" w325 {
                    tunnel: w327 -> [w342 w344]
                    tunnel: [w342 w343] -> w326
                    frame 0, Default {
                    }
                    frame 1099 {
                      n248 = call <vilib>:"Clear Errors.vi"("error in (no error)"=w344) -> ("error out"=w343:errorcluster)  [unwired: 6 in]
                    }
                  }
                }
                n249 = Close Reference(reference=w318) -> ()  [unwired: 1 in, 1 out]
              }
              frame Error {
                n250 = Close Reference(reference=w787) -> ()  [unwired: 1 in, 1 out]
              }
            }
            n251 = Bundle By Name(cluster=w305, "ReplacedVIsConPaneSize"=w303) -> (w304:T2)
          }
          frame "Save" {
            n252 = case shown="True" TRUE {
              tunnel: w794 -> [_ w804]
              tunnel: w793 -> [w795 w803]
              tunnel: [w795 w796] -> w792
              frame False {
              }
              frame True {
                w798 = FALSE  # IgnoreLibrarySaving
                n253 = invoke class="VI" method="Save.Instrument"(reference=w804, error in=w803) -> (reference out=w802:refnum<vi>, error out=w801:errorcluster)  [unwired: 4 in, 4 out]
                n254 = property class="VI"(reference=w802, error in=w801) -> (error out=w796:errorcluster, "Library"=w797:refnum<vi>)  [unwired: 1 out]
                n255 = Not A Number/Path/Refnum?(number/path/refnum=w797) -> (NaN/Path/Refnum?=w799:bool)
                n256 = Or(x=w799, y=w798) -> (x .or. y?=w800:bool)
                n257 = case shown="True" w800 {
                  tunnel: w797 -> [w806 w807]
                  frame False {
                    n258 = invoke class="Library" method="Save"(reference=w806) -> (reference out=w805:refnum<vi>)  [unwired: 3 in, 3 out]
                    n259 = Close Reference(reference=w805) -> ()  [unwired: 1 in, 1 out]
                  }
                  frame True {
                    n260 = Close Reference(reference=w807) -> ()  [unwired: 1 in, 1 out]
                  }
                }
              }
            }
          }
        }
        n261 = Equal?(x=w69, y="Exit") -> (x = y?=w72:bool)
        n262 = Select(t="Error", s=w68, f=w69) -> (s? t:f=w73:string)
      }
      n263 = Unbundle By Name(w11) -> ("ReplacedVIsConPaneSize"=w10:u32[])
    }
    frame Error {
    }
  }
  "error out" <- w8
  "ReplacedVIsConPaneSize" <- w1
  n264 = case shown="True" w3 {
    tunnel: w4 -> [_ w809]
    frame False {
    }
    frame True {
      n265 = Read from Text File(file (use dialog)=w809) -> (text=w812:string)  [unwired: 3 in, 3 out]
      n266 = Concatenate Strings(w812, ".\n" ("string")) -> (w810:string)
      n267 = stacked-sequence {
        tunnel: w810 -> [w815]
        tunnel: w809 -> [w814]
        frame #0 {
          n268 = Delete(path (use dialog)=w814) -> (deleted path=w813:path)  [unwired: 4 in, 2 out]
          n269 = Write to Text File(file (use dialog)=w813, text=w815) -> ()  [unwired: 2 in, 3 out]
        }
      }
    }
  }
